vi "Wrist Controller.vi"(8 "error in":errorcluster) -> ()   [LabVIEW 2018]
doc: "This VI executes continuously carrying out the current operation and responding to updates or new operations. It will often contain the timing or control code that is difficult to place directly in TeleOp. This VI generally opens all sensors and motors and isolates the rest of the robot code from knowing how the operations are carried out."
uses:
  <vilib>/Rock Robotics/WPI/Framework/Completion Status.ctl
  Wrist Setpoints.ctl
  Wrist Operations.ctl
  <vilib>/Rock Robotics/WPI/Solenoid/WPI_SolenoidChannel.ctl
  <vilib>/Rock Robotics/WPI/Solenoid/WPI_SolenoidValue.ctl
  <vilib>/Rock Robotics/WPI/Solenoid/WPI_SolenoidOpenDouble.vi
  <vilib>/Rock Robotics/WPI/Solenoid/WPI_SolenoidSetEnum.vi
  <vilib>/Rock Robotics/Network Tables/NT Write Boolean.vi
panel:
  in  "Interactive Values":T1
  out "Current\nCmd":string
  in  "Buttons":cluster{"Execute Cmd":bool, "Abort Cmd":bool}
  out "Command Timing":cluster{"Start Time (ms)":u32, "Iterations":i32}
  out "Status":T3
  # "Tip: It may be helpful to observe inputs and sensor values.\nYou may also want to display tuning or debugging controls."
  # "Interactive Command: You may fill in the settings for a command\nand schedule it with the Execute button. You can observe and abort\nany command while fine tuning the code for the controller."
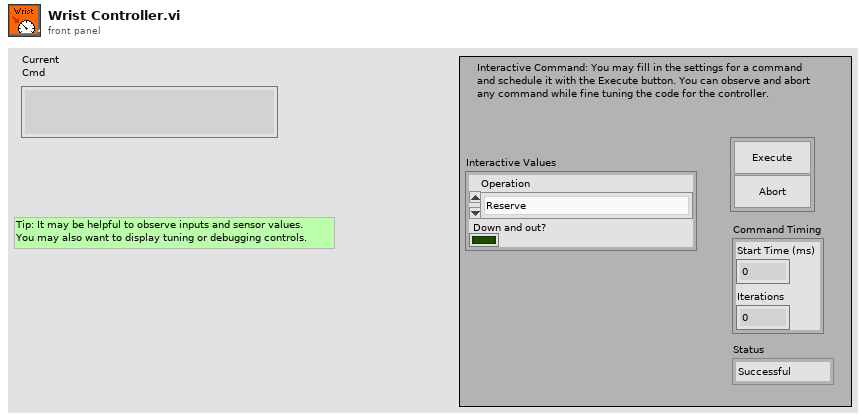
[diagram p1: front panel]
types:
  T1 = typedef "Wrist Setpoints.ctl" = cluster{"Operation":T2, "Down and out?":bool}
  T2 = typedef "Wrist Operations.ctl" = enum16{"Reserve", "Read Current", "SetPosition"}
  T3 = typedef "Completion Status.ctl" = enum16{"Successful", "Aborted", "Incomplete"}
  T4 = typedef "WPI_SolenoidChannel.ctl" = enum8{"Solenoid 0", "Solenoid 1", "Solenoid 2", "Solenoid 3", "Solenoid 4", "Solenoid 5", "Solenoid 6", "Solenoid 7", "Invalid"}
  T5 = typedef "WPI_SolenoidDevRef.ctl" = cluster{"DevStatus":errorcluster, "Pneumatics Control Module":u8, "Forward Solenoid Channel":T4, "Reverse Solenoid Channel":T4}
  T6 = typedef "Command Status Info.ctl" = cluster{"Name":string, "Status":T3, "notifier out":T7}
  T7 = typedef "Completion Notifier.ctl" = refnum<notifier>
  T8 = cluster{"Current Command":T1, "Command Timing":cluster{"Start Time (ms)":u32, "Iterations":i32}, "Command Arguments":cluster{"Command Info":T6, "Description":string, "Default Command":T1, "queue out":refnum<queue>, "Subsystem Name":string}}
  T9 = typedef "WPI_SolenoidValue.ctl" = enum16{"Off", "On", "Forward", "Reverse"}
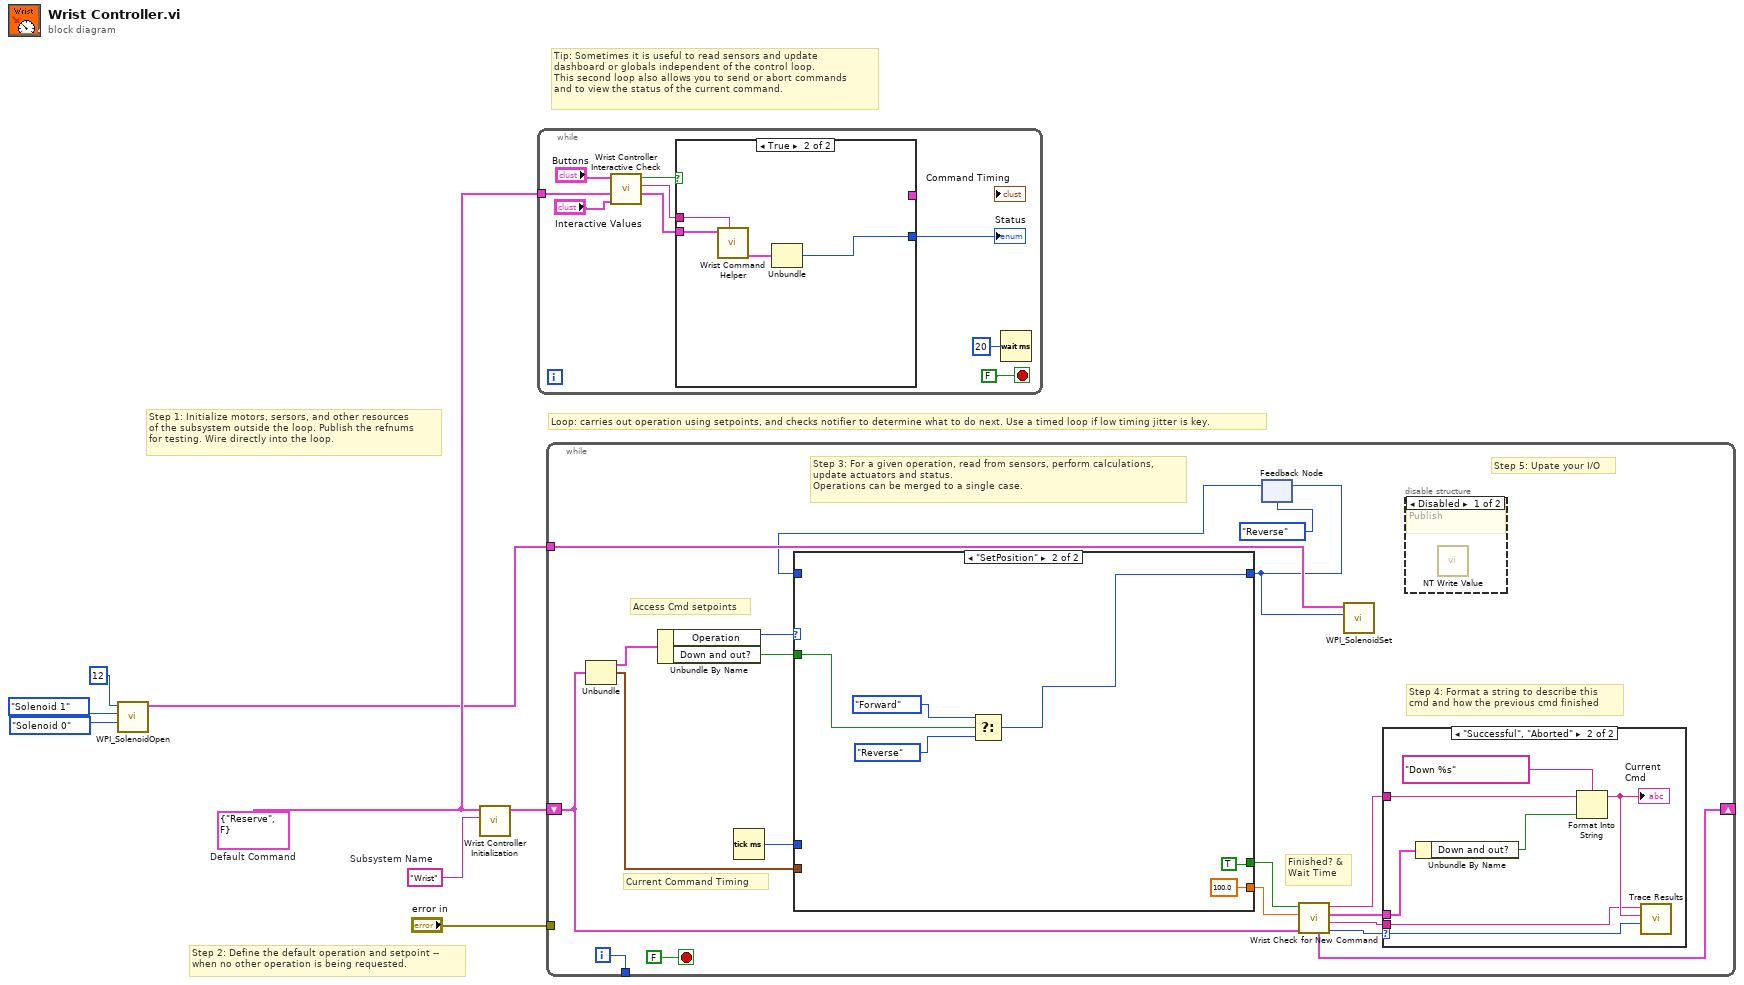
[diagram p0: block diagram]
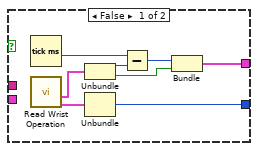
[diagram p2: hidden frame]
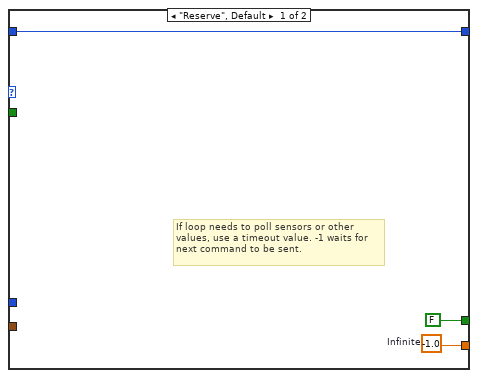
[diagram p5: hidden frame]
diagram:
  w5 = T1 {"Operation"=enum."Reserve", "Down and out?"=FALSE}  # Default Command
  w6 = "Wrist"  # Subsystem Name
  # "Tip: Sometimes it is useful to read sensors and update\ndashboard or globals independent of the control loop.\nThis second loop also allows you to send or abort commands\nand to view the status of the current command."
  # "Step 2: Define the default operation and setpoint --\nwhen no other operation is being requested."
  # "Step 1: Initialize motors, sersors, and other resources\nof the subsystem outside the loop. Publish the refnums\nfor testing. Wire directly into the loop."
  # "Loop: carries out operation using setpoints, and checks notifier to determine what to do next. Use a timed loop if low timing jitter is key."
  n1 = call-poly <vilib>:"WPI_SolenoidOpen.vi"("Reverse Solenoid Channel"=WPI_SolenoidChannel."Solenoid 0", "Forward Solenoid Channel"=WPI_SolenoidChannel."Solenoid 1", "Pneumatics Control Module (0)"=u8 12) -> ("SolenoidDevRef"=w1:T5)  [unwired: 7 in, 1 out]
  n2 = call "Wrist Controller Initialization.vi"("Subsystem Name"=w6, "Default Command"=w5) -> ("Current Command"=w7:T8)  [unwired: 9 in]
  n3 = while {
    tunnel: w5 -> [w14]
    stop <- FALSE stop-if-true
    n4 = call "Wrist Controller Interactive Check.vi"("Interactive Command in"="Interactive Values", "Default Command"=w14, "Buttons"="Buttons") -> ("Interactive Command out"=w11:T1, "Trace String"=w12:string, "Schedule"=w13:bool)  [unwired: 6 in]
    n5 = case shown="True" w13 {
      tunnel: [w25 w29] -> w10
      tunnel: w11 -> [_ w27]
      tunnel: [w21 _] -> _
      tunnel: w12 -> [_ w28]
      frame False {
        n6 = Tick Count (ms)() -> (millisecond timer value=w20:u32)
        n7 = call "Read Wrist Operation.vi"() -> ("Command Info"=w18:T6, "SubSystem Data"=w19:T1)  [unwired: 9 in, 1 out]
        n8 = Unbundle(w19) -> ("Operation"=w24:T2, "Down and out?"=w22:bool)
        n9 = Unbundle(w18) -> ("Status"=w25:T3)  [unwired: 2 out]
        n10 = Subtract(x=w20, y=w24) -> (x-y=w23:u32)
        n11 = Bundle(w23, "Down and out?"=w22) -> (w21:cluster{u32, "Down and out?":bool})  [unwired: 1 in]
      }
      frame True {
        n12 = call "Wrist Command Helper.vi"("Description"=w28, "SubSystem Data"=w27) -> ("Command Info Out"=w26:T6)  [unwired: 7 in, 2 out]
        n13 = Unbundle(w26) -> ("Status"=w29:T3)  [unwired: 2 out]
      }
    }
    "Status" <- w10
    n14 = Wait (ms)(milliseconds to wait=u32 20) -> ()  [unwired: 1 out]
  }
  n15 = while {
    shift-right: [w42] -> _
    shift-left: w7 -> [w35]
    tunnel: [w47] -> _
    tunnel: "error in" -> [_]
    tunnel: w1 -> [w33]
    i -> [w47]
    stop <- FALSE stop-if-true
    # "Step 5: Upate your I/O"
    # "Step 4: Format a string to describe this\ncmd and how the previous cmd finished"
    # "Current Command Timing"
    # "Access Cmd setpoints"
    # "Finished? &\nWait Time"
    # "Step 3: For a given operation, read from sensors, perform calculations,\nupdate actuators and status.\nOperations can be merged to a single case."
    n16 = Unbundle(w35) -> ("Current Command"=w46:T1, "Command Timing"=w43:cluster{"Start Time (ms)":u32, "Iterations":i32})  [unwired: 1 out]
    n17 = Unbundle By Name(w46) -> ("Operation"=w45:T2, "Down and out?"=w34:bool)
    n18 = Tick Count (ms)() -> (millisecond timer value=w44:u32)
    n19 = feedback #1(WPI_SolenoidValue."Reverse" ("Value")) -> (w31:T9)
    n20 = case shown="\"SetPosition\"" w45 {
      tunnel: [w58 100.0 ("Infinite")] -> w40
      tunnel: [FALSE ("ignore previous (F)") TRUE] -> w41
      tunnel: w43 -> [_ _]
      tunnel: w44 -> [_ _]
      tunnel: w34 -> [_ w64]
      tunnel: [w56 w61] -> w30
      tunnel: w31 -> [w56 _]
      frame "Reserve", Default {
        w58 = -1.0  # Infinite
        # "If loop needs to poll sensors or other\nvalues, use a timeout value. -1 waits for\nnext command to be sent."
      }
      frame "SetPosition" {
        n21 = Select(t=WPI_SolenoidValue."Forward" ("Value"), s=w64, f=WPI_SolenoidValue."Reverse" ("Value")) -> (s? t:f=w61:T9)
      }
    }
    n22 = feedback-in #1(w30) -> ()
    n23 = call "Wrist Check for New Command.vi"("Current Command"=w35, "Wait time (ms)"=w40, "Finished?"=w41) -> ("Completion"=w36:T3, "Subsystem Name"=w37:string, "Current Command"=w38:T1, "Initial Trace String"=w39:string, "NextCommand"=w42:T8)  [unwired: 4 in]
    n24 = call-poly <vilib>:"WPI_SolenoidSet.vi"("Value"=w30, "SolenoidDevRef"=w33) -> ()  [unwired: 8 in, 2 out]
    n25 = case shown="\"Successful\", \"Aborted\"" w36 {
      selector: w36 -> [_ w55]
      tunnel: w39 -> [_ w52]
      tunnel: w38 -> [_ w53]
      tunnel: w37 -> [_ w50]
      frame "Incomplete", Default {
        # "Continuing current command"
      }
      frame "Successful", "Aborted" {
        # "Report and setup for next command"
        n26 = Unbundle By Name(w53) -> ("Down and out?"=w49:bool)
        n27 = Format Into String(format string="Down %s", initial string=w52, w49) -> (resulting string=w51:string)  [unwired: 1 in, 1 out]
        "Current\nCmd" <- w51
        n28 = call <vilib>:"Trace Results.vi"("Status of previous command"=w55, "Description"=w51, "Subsystem"=w50) -> ()  [unwired: 9 in]
      }
    }
    n29 = disable-structure shown="Disabled" {
      frame Disabled {
        # "Publish"
        n30 = call-poly <vilib>:"NT Write Value.vi"() -> ()  [unwired: 11 in, 1 out]
      }
      frame Enabled {
      }
    }
  }
